vi "basculaRS_SubVI.vi"() -> ()   [LabVIEW 2019]
panel:
  out ".not. (x .or. y)? 2":bool
  out ".not. (x .or. y)?":bool
  in  "y":bool
  in  "x":bool
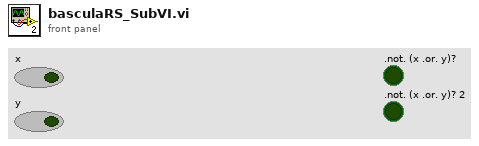
[diagram p1: front panel]
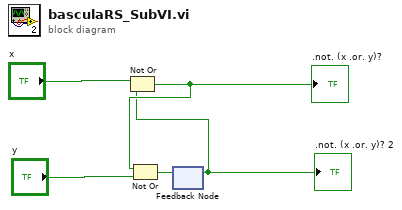
[diagram p0: block diagram]
diagram:
  n1 = feedback #1() -> (w1:bool)  [unwired: 1 in]
  ".not. (x .or. y)? 2" <- w1
  n2 = Not Or(1:w1, 2:"x") -> (0:w3:bool)
  ".not. (x .or. y)?" <- w3
  n3 = Not Or(1:"y", 2:w3) -> (0:w2:bool)
  n4 = feedback-in #1(w2) -> ()
